vi "Launch Main Program.vi"   [LabVIEW 2013]
uses:
  Tesla Tester GUI/Tesla Tester GUI_Actor/Tesla Tester GUI.lvclass
  <vilib>/ActorFramework/Message Queue/Message Queue.lvclass/Message Queue.ctl
  <vilib>/ActorFramework/Actor/Actor.lvclass
  <vilib>/ActorFramework/Message Queue/Message Queue.lvclass
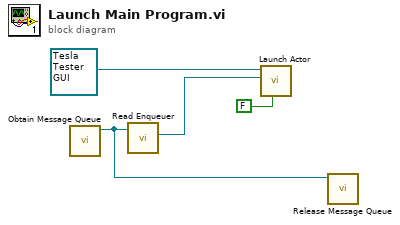
[diagram p0: block diagram]
diagram:
  n1 = call <vilib>:"Obtain Message Queue.vi"() -> ("Message Queue"=w2:refnum<class "Message Queue.lvclass">)  [unwired: 10 in, 1 out]
  n2 = call <vilib>:"Read Enqueuer.vi"("Message Queue"=w2) -> ("Message Enqueuer"=w3:refnum<class "Message Enqueuer.lvclass">)  [unwired: 10 in]
  n3 = call <vilib>:"Launch Actor.vi"("Open Actor Core front panel? (F)"=FALSE, "Actor-to-Caller Enqueuer"=w3, "Actor"=refnum<class "Tesla Tester GUI.lvclass"> refnum ("Tesla Tester GUI.lvlib:Tesla Tester GUI")) -> ()  [unwired: 7 in, 2 out]
  n4 = call <vilib>:"Release Message Queue.vi"("Message Queue"=w2) -> ()  [unwired: 9 in, 2 out]
